vi "ClassPanel.vi"(8 "error in (no error)":errorcluster caption="entrée d'erreur (pas d'erreur)", 11 "SR400.lvclass":refnum<class "SR400.lvclass">) -> (0 "error out":errorcluster caption="sortie d'erreur", 3 "SR400.lvclass Out":refnum<class "SR400.lvclass">)   [LabVIEW 2012, in "SR400.lvclass"]
uses:
  SR400.lvclass
  BaseDevice/Accessor/GetClassEvent.vi
  <vilib>/Analysis/baseanly.llb/Mean (DBL).vi
  <vilib>/Analysis/NI_AALBase.lvlib
panel:
  out "Mode":u16(ring) items=["A,B for T Preset", "A-B for T Preset", "A+B for T Preset", "A for B preset"]
  in  "CounterPresT":dbl=0.001 caption="Counter T Preset (s)" min=1e-07 max=90000.0 step=1e-07 format="%#.7g"
  in  "Dwell time":dbl=6.0 caption="\"Dwell Time\" (s)" min=0.002 max=6.0 step=0.001
  out "Comptes":dbl[](array[numeric])
  in  "Compteur":u16(ring) items=["A", "B", "A+B"]
  out "ACQ":bool
  in  "Stop":bool
  out "Count":dbl caption="Compte Moy (photon)"
  in  "MiseAJour":bool
  in  "NbPeriod":i32=1 caption="Nb de périodes" min=1 max=1000 step=1
  out "Init Program":bool
  # "SR400 Photon Counter Panel"
  # "this MUST labeled with class name"
  # "this MUST be present and labeled \"Stop\""
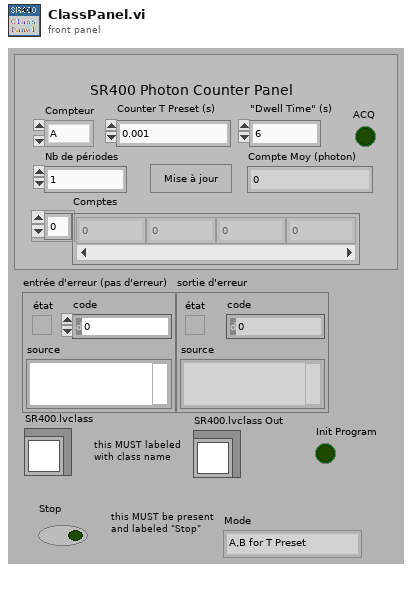
[diagram p1: front panel]
types:
  T1 = enum16{"All", "Mode", "T Preset", "B Preset", "Dwell", "NbPeriod"}
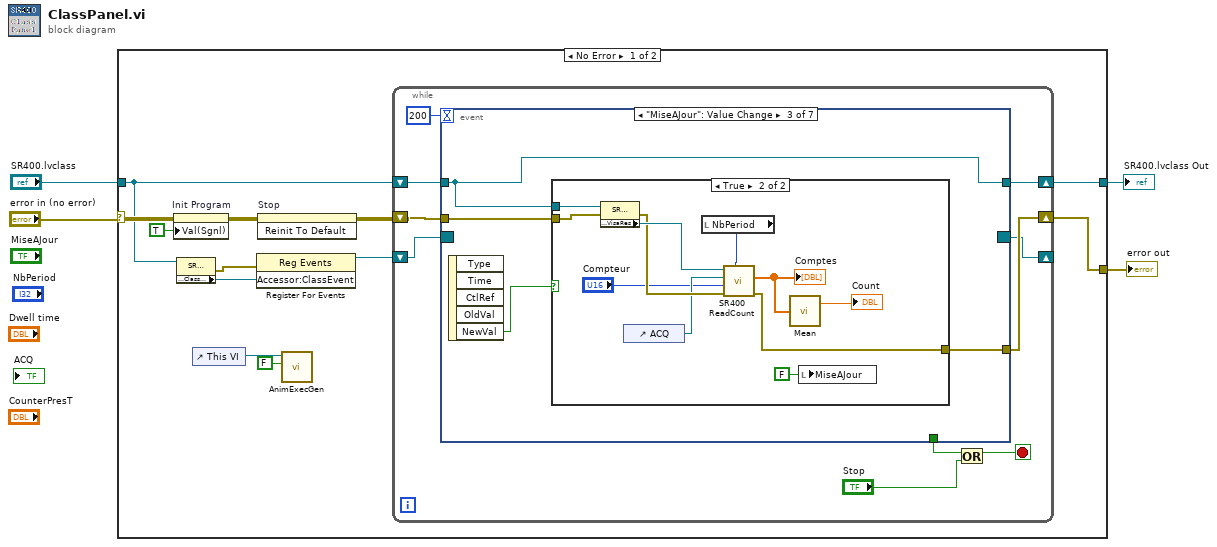
[diagram p0: block diagram]
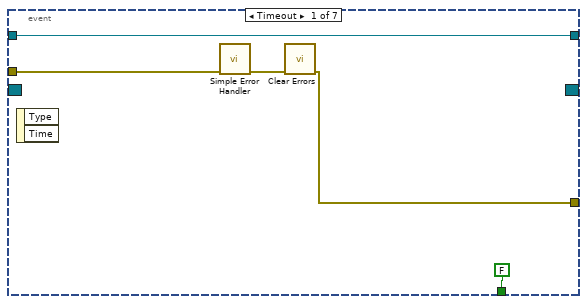
[diagram p2: hidden frame]
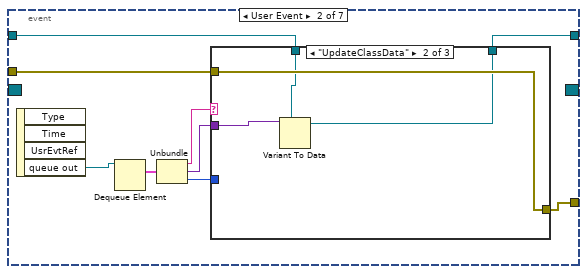
[diagram p3: hidden frame]
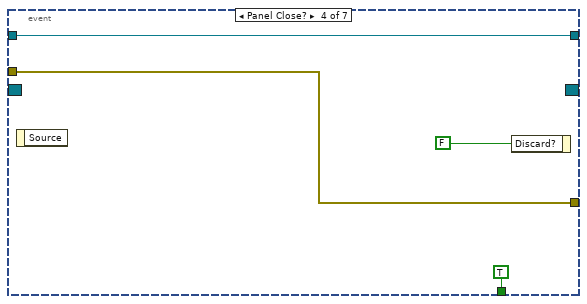
[diagram p7: hidden frame]
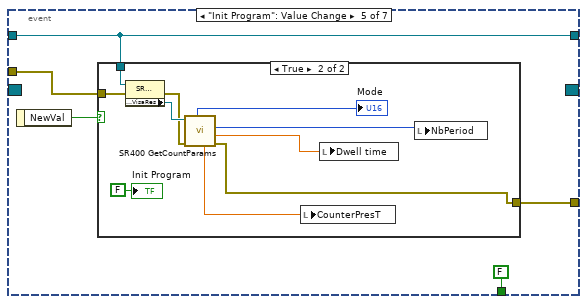
[diagram p8: hidden frame]
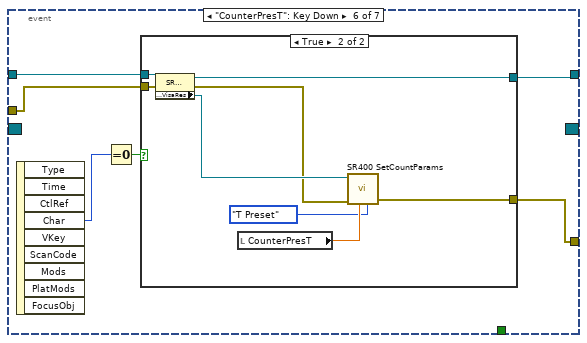
[diagram p10: hidden frame]
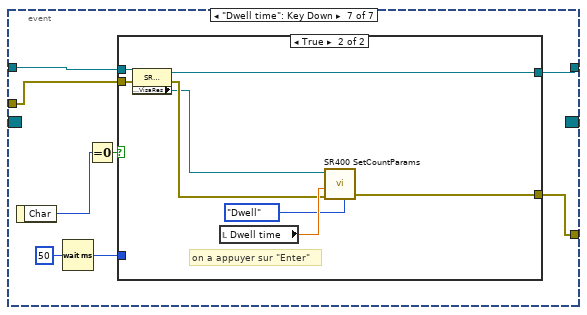
[diagram p12: hidden frame]
diagram:
  n1 = case shown="No Error" "error in (no error)" {
    selector: "error in (no error)" -> [w13 w120]
    tunnel: [w16 w120] -> w3
    tunnel: "SR400.lvclass" -> [w8 w119]
    tunnel: [w14 w119] -> w1
    frame No Error {
      n2 = property on="Init Program" class="Bool (strict)"(error in=w13, "Val(Sgnl)"=TRUE ("Valeur (Signalisation)")) -> (error out=w12:errorcluster)  [unwired: 1 in, 1 out]
      n3 = property class="SR400.lvclass"(reference=w8) -> (error out=w10:errorcluster, "Accessor:ClassEvent"=w9:refnum<user-event>)  [unwired: 1 in, 1 out]
      n4 = control-ref of="This VI"() -> (w5:refnum<vi>)
      n5 = register-events(error in=w10, w9) -> (reference out=w7:refnum<event-registration>)  [unwired: 1 in, 1 out]
      n6 = invoke on="Stop" class="Bool (strict)" method="Reinit To Default"(error in=w12) -> (error out=w11:errorcluster)  [unwired: 2 in, 2 out]
      n7 = call <userlib>:"AnimExecGen.vi"("Animer l'exécution ?"=FALSE, "ViRef"=w5) -> ()  [unwired: 9 in, 1 out]
      n8 = while {
        shift-right: [w24] -> w16
        shift-left: w11 -> [w25]
        shift-right: [w21] -> w14
        shift-left: w8 -> [w23]
        shift-right: [w17] -> _
        shift-left: w7 -> [w18]
        stop <- w20 stop-if-true
        n9 = event shown="[2] \"MiseAJour\": Value Change" {
          selector: w18 -> [_ _ _ _ _ _ _]
          dyn-events: [_ _ _ _ _ _ _] -> w17
          timeout: 200 -> [_ _ _ _ _ _ _]
          tunnel: w25 -> [w29 w39 w50 w66 w70 w88 w106]
          tunnel: [w27 w33 w49 w66 w72 w87 w105] -> w24
          tunnel: w23 -> [w30 w40 w51 w65 w69 w90 w108]
          tunnel: [FALSE _ _ TRUE FALSE _ _] -> w22
          tunnel: [w30 w32 w51 w65 w69 w89 w107] -> w21
          event Timeout {
            n10 = event-data() -> ()  [unwired: 1 in, 2 out]
            n11 = call <vilib>:"Simple Error Handler.vi"("error in (no error)"=w29) -> ("error out"=w28:errorcluster)  [unwired: 4 in, 4 out]
            n12 = call <vilib>:"Clear Errors.vi"("error in (no error)"=w28) -> ("error out"=w27:errorcluster)  [unwired: 6 in]
          }
          event User Event {
            n13 = event-data() -> ("queue out"=w37:refnum<queue>)  [unwired: 1 in, 3 out]
            n14 = Dequeue Element(queue=w37) -> (element=w38:cluster{"Message":string, "Data":variant, i32})  [unwired: 2 in, 3 out]
            n15 = Unbundle(w38) -> ("Message"=w36:string, "Data"=w35:variant, w34:i32)
            n16 = case shown="\"UpdateClassData\"" w36 {
              tunnel: w39 -> [w42 w46 w47]
              tunnel: w35 -> [_ w45 _]
              tunnel: w40 -> [w41 w44 w48]
              tunnel: [w41 w43 w48] -> w32
              tunnel: [w42 w46 w47] -> w33
              tunnel: w34 -> [_ _ _]
              frame Default {
              }
              frame "UpdateClassData" {
                n17 = Variant To Data(type=w44, Variant=w45) -> (data=w43:refnum<class "SR400.lvclass">)  [unwired: 1 in, 1 out]
              }
              frame "MeasDone" {
              }
            }
          }
          event "MiseAJour": Value Change {
            n18 = event-data() -> ("NewVal"=w52:bool)  [unwired: 1 in, 4 out]
            n19 = case shown="True" w52 {
              tunnel: w51 -> [_ w64]
              tunnel: w50 -> [w53 w62]
              tunnel: [w53 w60] -> w49
              frame False {
              }
              frame True {
                n20 = property class="SR400.lvclass"(reference=w64, error in=w62) -> (error out=w61:errorcluster, "Accessor:VisaRes"=w63:refnum<visa-resource-name>)  [unwired: 1 out]
                n21 = control-ref of="ACQ"() -> (w57:refnum<vi>)
                n22 = local read "NbPeriod"() -> (w58:i32)
                n23 = call <userlib>:"SR400 ReadCount.vi"("Nb de période"=w58, "error in (no error)"=w61, "Compteur"="Compteur", "AcqRef"=w57, "VISA Port In"=w63) -> ("error out"=w60:errorcluster, "Données"=w55:dbl[])  [unwired: 3 in, 2 out]
                "Comptes" <- w55
                n24 = call-poly <vilib>:"Mean.vi"("X"=w55) -> ("mean"=→"Count":dbl)  [unwired: 1 out]
                n25 = local write "MiseAJour"(FALSE ("MiseAJour")) -> ()
              }
            }
          }
          event Panel Close? {
            n26 = event-data() -> ()  [unwired: 1 in, 1 out]
            n27 = event-data("Discard?"=FALSE ("Rejeter ?")) -> ()  [unwired: 1 in, 1 out]
          }
          event "Init Program": Value Change {
            n28 = event-data() -> ("NewVal"=w73:bool)  [unwired: 1 in]
            n29 = case shown="True" w73 {
              tunnel: [w74 w77] -> w72
              tunnel: w70 -> [w74 w83]
              tunnel: w69 -> [_ w82]
              frame False {
              }
              frame True {
                n30 = property class="SR400.lvclass"(reference=w82, error in=w83) -> (error out=w80:errorcluster, "Accessor:VisaRes"=w81:refnum<visa-resource-name>)  [unwired: 1 out]
                n31 = call <userlib>:"SR400 GetCountParams.vi"("error in (no error)"=w80, "VISA Port In"=w81) -> ("error out"=w77:errorcluster, "Dwell time"=w78:dbl, "Nb de période"=w79:i32, "CounterPresT"=w76:dbl, "Mode"=→"Mode":u16)  [unwired: 3 in, 2 out]
                n32 = local write "CounterPresT"(w76) -> ()
                n33 = local write "Dwell time"(w78) -> ()
                n34 = local write "NbPeriod"(w79) -> ()
                "Init Program" <- FALSE
              }
            }
          }
          event "CounterPresT": Key Down {
            n35 = event-data() -> ("Char"=w85:i16)  [unwired: 1 in, 8 out]
            n36 = Equal To 0?(x=w85) -> (x = 0?=w86:bool)
            n37 = case shown="True" w86 {
              tunnel: w90 -> [w92 w100]
              tunnel: [w92 w99] -> w89
              tunnel: w88 -> [w91 w98]
              tunnel: [w91 w97] -> w87
              frame False {
              }
              frame True {
                n38 = property class="SR400.lvclass"(reference=w100, error in=w98) -> (reference out=w99:refnum<class "SR400.lvclass">, error out=w93:errorcluster, "Accessor:VisaRes"=w95:refnum<visa-resource-name>)
                n39 = local read "CounterPresT"() -> (w96:dbl)
                n40 = call <userlib>:"SR400 SetCountParams.vi"("Operation"=T1."T Preset", "Counter T Preset (s)"=w96, "error in (no error)"=w93, "VISA Port In"=w95) -> ("error out"=w97:errorcluster)  [unwired: 5 in, 1 out]
              }
            }
          }
          event "Dwell time": Key Down {
            n41 = event-data() -> ("Char"=w104:i16)  [unwired: 1 in]
            n42 = Wait (ms)(milliseconds to wait=u32 50) -> (millisecond timer value=w102:u32)
            n43 = Equal To 0?(x=w104) -> (x = 0?=w103:bool)
            n44 = case shown="True" w103 {
              tunnel: w108 -> [w110 w118]
              tunnel: [w110 w117] -> w107
              tunnel: w106 -> [w109 w116]
              tunnel: [w109 w115] -> w105
              tunnel: w102 -> [_ _]
              frame False {
              }
              frame True {
                # "on a appuyer sur \"Enter\""
                n45 = property class="SR400.lvclass"(reference=w118, error in=w116) -> (reference out=w117:refnum<class "SR400.lvclass">, error out=w113:errorcluster, "Accessor:VisaRes"=w112:refnum<visa-resource-name>)
                n46 = local read "Dwell time"() -> (w114:dbl)
                n47 = call <userlib>:"SR400 SetCountParams.vi"("Operation"=T1."Dwell", "error in (no error)"=w113, "Dwell time"=w114, "VISA Port In"=w112) -> ("error out"=w115:errorcluster)  [unwired: 5 in, 1 out]
              }
            }
          }
        }
        n48 = Or(x=w22, y="Stop") -> (x .or. y?=w20:bool)
      }
    }
    frame Error {
    }
  }
  "error out" <- w3
  "SR400.lvclass Out" <- w1
